vi "Read Default From File.vi"(8 "error in (no error)":errorcluster, 9 "Name":string, 10 "Path":path, 11 "Dot Settings in":refnum<class "Dot Settings.lvclass">) -> (0 "error out":errorcluster, 3 "Dot Settings out":refnum<class "Dot Settings.lvclass">)   [LabVIEW 2019, in "Dot Settings.lvclass"]
uses:
  Dot Settings.lvclass
  ObjectSettings/ObjectSettings.lvclass
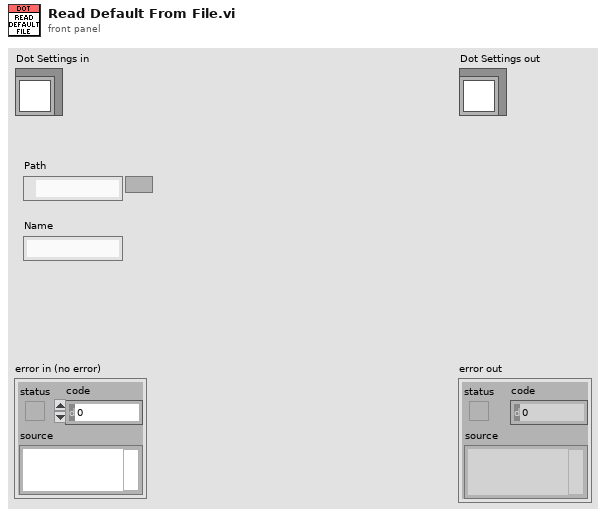
[diagram p1: front panel]
types:
  T1 = typedef "Dot Settings.lvclass/Default Dot Cluster.ctl" = cluster{"Action":T2, "Dot KVPs":cluster{"Key":string, "Value":string}[]}
  T2 = typedef "Dot Settings.lvclass/Action.ctl" = enum16{"IV", "QD"}
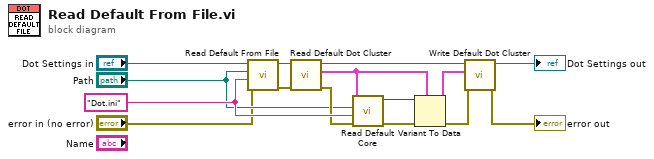
[diagram p0: block diagram]
diagram:
  w13 = "Dot.ini"
  n1 = call-parent "Read Default From File.vi"("error in (no error)"="error in (no error)", "Name"=w13, "Path"="Path", "ObjectSettings in"="Dot Settings in") -> ("error out"=w9:errorcluster, "ObjectSettings out"=w11:refnum<class "Dot Settings.lvclass">)  [unwired: 6 in]
  n2 = call "Read Default Dot Cluster.vi"("error in (no error)"=w9, "Dot Settings in"=w11) -> ("error out"=w8:errorcluster, "Default Dot"=w10:T1, "Dot Settings out"=w7:refnum<class "Dot Settings.lvclass">)  [unwired: 7 in]
  n3 = call "Read Default Core.vi"("error in (no error)"=w8, "Name"=w13, "Path"="Path", "Cluster In"=w10) -> ("error out"=w15:errorcluster, "Cluster Out"=w14:variant)  [unwired: 6 in]
  n4 = Variant To Data(error in=w15, type=w10, Variant=w14) -> (data=w5:T1, error out=w2:errorcluster)
  n5 = call "Write Default Dot Cluster.vi"("error in (no error)"=w2, "Default Dot"=w5, "Dot Settings in"=w7) -> ("error out"=→"error out":errorcluster, "Dot Settings out"=→"Dot Settings out":refnum<class "Dot Settings.lvclass">)  [unwired: 7 in]
